vi "AppendData.vi"(8 "Error In":errorcluster, 9 "Name":string, 10 "Data":dbl[](array[numeric]), 11 "Folder":path) -> (0 "Error Out":errorcluster, 3 "File Path Control out":path)   [LabVIEW 2015]
panel:
  out "appended path":path
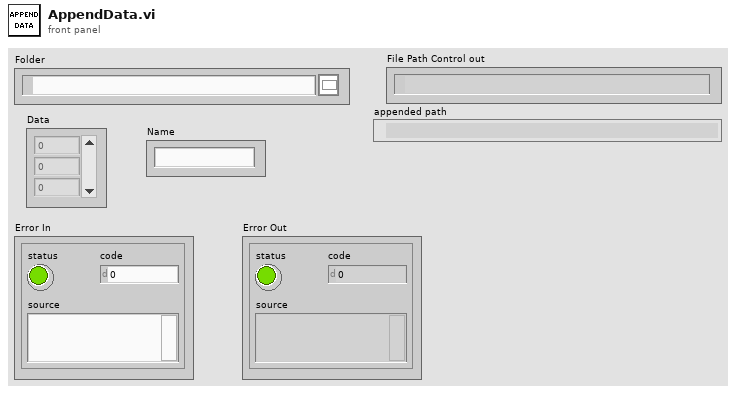
[diagram p1: front panel]
types:
  T1 = enum16{"open", "replace", "create", "open or create", "replace or create", "replace or create with confirmation"}
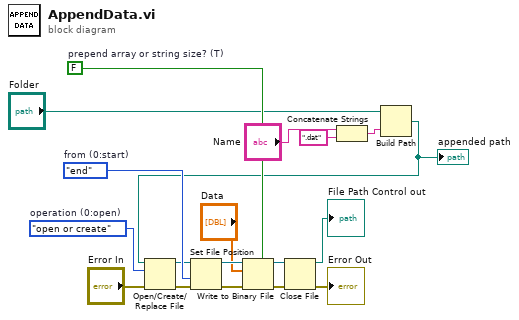
[diagram p0: block diagram]
diagram:
  w7 = FALSE  # prepend array or string size? (T)
  w16 = enum16{"start", "end", "current"}."end"  # from (0:start)
  w18 = T1."open or create"  # operation (0:open)
  n1 = Concatenate Strings("Name", ".dat" ("string")) -> (w3:string)
  n2 = Build Path(base path="Folder", name or relative path=w3) -> (appended path=w1:path)
  "appended path" <- w1
  n3 = Open/Create/Replace File(file path (use dialog)=w1, error in="Error In", operation (0:open)=w18) -> (refnum out=w14:refnum<file>, error out=w15:errorcluster)  [unwired: 3 in, 1 out]
  n4 = Set File Position(refnum=w14, from (0:start)=w16, error in=w15) -> (refnum out=w13:refnum<file>, error out=w12:errorcluster)  [unwired: 1 in]
  n5 = Write to Binary File(file (use dialog)=w13, data="Data", error in=w12, 5:w7) -> (refnum out=w8:refnum<file>, error out=w10:errorcluster)  [unwired: 2 in, 1 out]
  n6 = Close File(refnum=w8, error in=w10) -> (path=→"File Path Control out":path, error out=→"Error Out":errorcluster)
